vi "Inst.Krohn-Hite-7008.handleGetCommand.vi"(8 "error in (no error)":errorcluster, 9 "Data":variant, 10 "Command in":string, 11 "Inst.Krohn-Hite-7008 in":refnum<class "Inst.Krohn-Hite-7008.lvclass">) -> (0 "error out":errorcluster, 1 "Data out":variant, 2 "Command out":string, 3 "Inst.Krohn-Hite-7008 out":refnum<class "Inst.Krohn-Hite-7008.lvclass">)   [LabVIEW 2019, in "Inst.Krohn-Hite-7008.lvclass"]
uses:
  Inst.Krohn-Hite-7008.lvclass
  Inst.Krohn-Hite-7008.lvclass/Inst.Krohn-Hite-7008.ctl
  Typedefs/Inst.Krohn-Hite-7008.ProtectedCommands--Enum.ctl
  Typedefs/getChannelRequest--Cluster.ctl
  KH7008/typedefs/channel--numeric.ctl
  a0eabf90-b4d9-4584-866f-9f1db62b2114.vi
  a0eabf90-b4d9-4584-866f-9f1db62b2114.vi/c33843f7-451f-4e2e-a4e3-fc07b03aa2e1.vi
  a0eabf90-b4d9-4584-866f-9f1db62b2114.vi/53209b5d-dba8-4aeb-859b-6a1b8073345c.vi
  <vilib>/Utility/Data Type/Get Type Information.vi
  <vilib>/JDP Science/JSONtext/JSON text to Variant.vi
  <vilib>/JDP Science/JSONtext/LVClass Serializer/JSONtext LVClass Serializer.lvclass
  KH7008/KH7008.lvlib
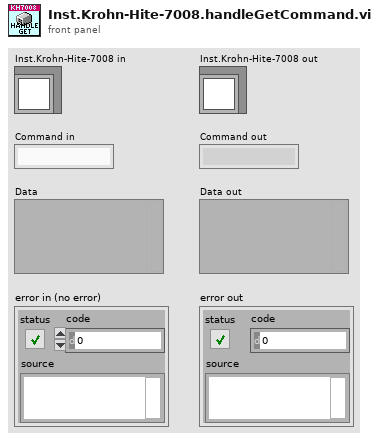
[diagram p1: front panel]
types:
  T1 = typedef "Inst.Krohn-Hite-7008.lvclass/Inst.Krohn-Hite-7008.ProtectedCommands--Enum.ctl" = enum16{"Update allChannelProperties", "Update device", "Set SR"}
  T2 = typedef "Inst.Krohn-Hite-7008.lvclass/getChannelRequest--Cluster.ctl" = cluster{"channel":T3}
  T3 = typedef "KH7008.lvlib/channel--numeric.ctl" = u16
  T4 = typedef "KH7008.lvlib/allChannelProperties--Array.ctl" = T5[]
  T5 = typedef "KH7008.lvlib/channelProperties--Cluster.ctl" = cluster{"channel":T3, "gain":T6, "input":T7, "shunt":T8, "couple":T9, "filter":T10}
  T6 = typedef "KH7008.lvlib/gain--enum.ctl" = enum16{"1x", "10x", "100x", "1000x"}
  T7 = typedef "KH7008.lvlib/input--enum.ctl" = enum16{"OFF", "SE+", "SE-", "DIFF"}
  T8 = typedef "KH7008.lvlib/shunt--enum.ctl" = enum16{"Open", "50", "500", "5k", "50k", "10M"}
  T9 = typedef "KH7008.lvlib/couple--enum.ctl" = enum16{"AC", "DC"}
  T10 = typedef "KH7008.lvlib/filter--enum.ctl" = enum16{"OFF", "ON"}
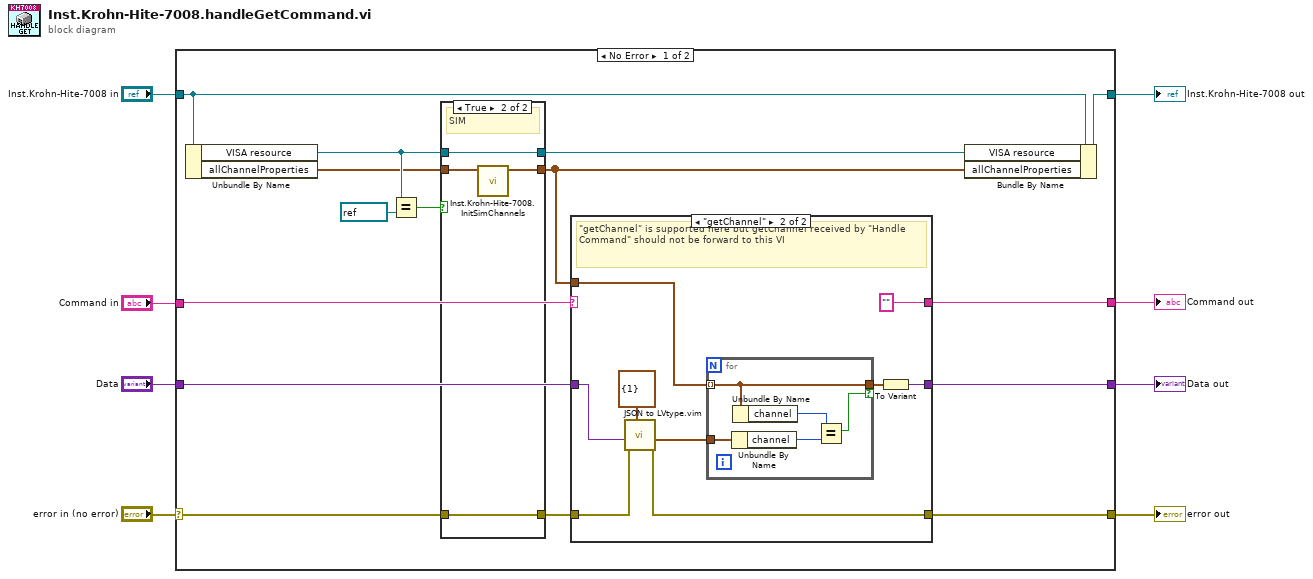
[diagram p0: block diagram]
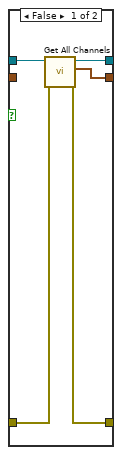
[diagram p2: hidden frame]
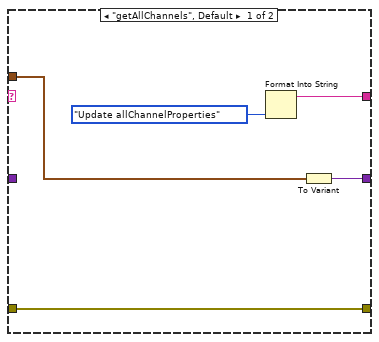
[diagram p3: hidden frame]
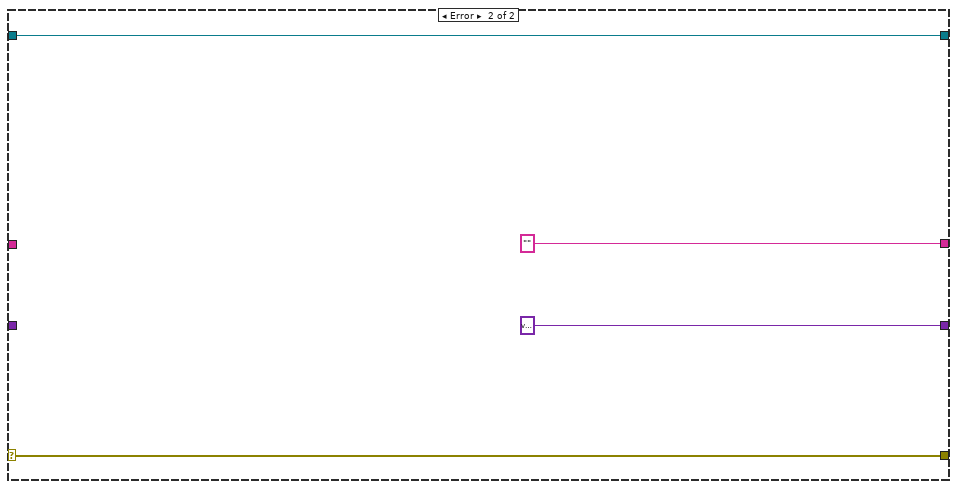
[diagram p4: hidden frame]
diagram:
  n1 = case shown="No Error" "error in (no error)" {
    selector: "error in (no error)" -> [w23 w55]
    tunnel: [w22 w55] -> w7
    tunnel: [w16 w54] -> w6
    tunnel: "Inst.Krohn-Hite-7008 in" -> [w18 w54]
    tunnel: [w12 "" ("Command")] -> w4
    tunnel: [w13 variant ("Variant")] -> w3
    tunnel: "Command in" -> [w21 _]
    tunnel: "Data" -> [w17 _]
    frame No Error {
      n2 = Unbundle By Name(w18) -> ("VISA resource"=w20:refnum<visa-resource-name>, "allChannelProperties"=w14:T4)
      n3 = Equal?(x=w20, y=refnum<visa-resource-name> "sim") -> (x = y?=w9:bool)
      n4 = case shown="True" w9 {
        tunnel: [w28 w32] -> w19
        tunnel: w23 -> [w27 w31]
        tunnel: [w26 w30] -> w15
        tunnel: [w25 w31] -> w11
        tunnel: w20 -> [w24 w32]
        tunnel: w14 -> [_ w29]
        frame False {
          n5 = call "Get All Channels.vi"("error in (no error)"=w27, "VISA Refnum in"=w24) -> ("error out"=w25:errorcluster, "allChannelProperties"=w26:T4, "VISA Refnum out"=w28:refnum<visa-resource-name>)  [unwired: 7 in]
        }
        frame True {
          # "SIM"
          n6 = call "Inst.Krohn-Hite-7008.InitSimChannels.vi"("allChannelProperties"=w29) -> ("allChannelProperties"=w30:T4)  [unwired: 10 in]
        }
      }
      n7 = case shown="\"getChannel\"" w21 {
        tunnel: w15 -> [w33 w41]
        tunnel: [w37 w44] -> w13
        tunnel: w17 -> [_ w45]
        tunnel: w11 -> [w34 w43]
        tunnel: [w34 w38] -> w22
        tunnel: [w35 ""] -> w12
        frame "getAllChannels", Default {
          n8 = Format Into String(Inst.Krohn-Hite-7008.ProtectedCommands--Enum."Update allChannelProperties" ("Commands")) -> (resulting string=w35:string)  [unwired: 3 in, 1 out]
          n9 = To Variant(anything=w33) -> (Variant=w37:variant)
        }
        frame "getChannel" {
          # "\"getChannel\" is supported here but getChannel received by \"Handle Command\" should not be forward to this VI"
          n10 = call "JSON to LVtype.vim"("type"=T2 {"channel"=1} ("getChannelRequest"), "error in (no error)"=w43, "JSON Data in"=w45) -> ("error out"=w38:errorcluster, "Data out"=w42:T2)  [unwired: 7 in]
          n11 = for {
            tunnel: w41 -> [w50] mode=indexing
            tunnel: [w50] -> w39 if=w49
            tunnel: w42 -> [w48]
            n12 = Unbundle By Name(w48) -> ("channel"=w47:T3)
            n13 = Unbundle By Name(w50) -> ("channel"=w51:T3)
            n14 = Equal?(x=w51, y=w47) -> (x = y?=w49:bool)
          }
          n15 = To Variant(anything=w39) -> (Variant=w44:variant)
        }
      }
      n16 = Bundle By Name(cluster=w18, "VISA resource"=w19, "allChannelProperties"=w15) -> (w16:refnum<class "Inst.Krohn-Hite-7008.lvclass">)
    }
    frame Error {
    }
  }
  "error out" <- w7
  "Inst.Krohn-Hite-7008 out" <- w6
  "Command out" <- w4
  "Data out" <- w3
